vi "Compensation_mA_100mA_Peaks.vi"(11 "Waveform in":waveform(sgl)) -> (3 "Waveform out":waveform(sgl))   [LabVIEW 2017]
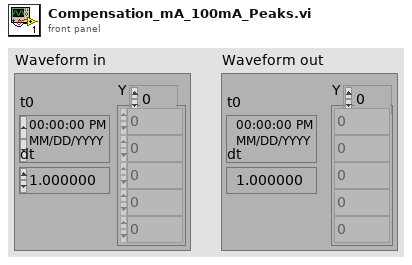
[diagram p1: front panel]
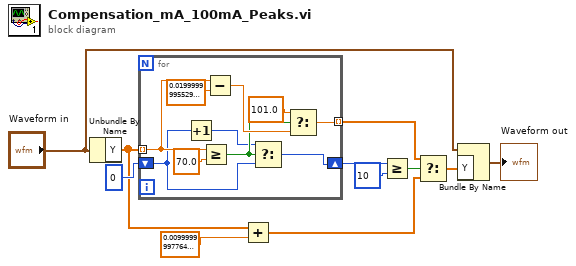
[diagram p0: block diagram]
diagram:
  n1 = Unbundle By Name("Waveform in") -> ("Y"=w3:sgl[])
  n2 = for {
    tunnel: w3 -> [w18] mode=indexing
    tunnel: [w20] -> w5 mode=indexing
    shift-right: [w13] -> w8
    shift-left: 0 -> [w12]
    n3 = Increment(x=w12) -> (x+1=w14:i32)
    n4 = Greater Or Equal?(x=w18, y=sgl 70.0) -> (x >= y?=w15:bool)
    n5 = Subtract(x=w18, y=sgl 0.02) -> (x-y=w16:sgl)
    n6 = Select(t=w14, s=w15, f=w12) -> (s? t:f=w13:i32)
    n7 = Select(t=sgl 101.0, s=w15, f=w16) -> (s? t:f=w20:sgl)
  }
  n8 = Add(x=w3, y=sgl 0.01) -> (x+y=w1:sgl[])
  n9 = Greater Or Equal?(x=w8, y=10) -> (x >= y?=w6:bool)
  n10 = Select(t=w5, s=w6, f=w1) -> (s? t:f=w4:sgl[])
  n11 = Bundle By Name(cluster="Waveform in", "Y"=w4) -> (→"Waveform out":waveform(sgl))
